vi "iWorx Drop Counter SubVI.vi"(4 "minimum drop delta (.05s)":dbl=0.01, 6 "# of Timestamps to store":i32=10, 7 "Reset count (f)":bool, 10 "Threshold (0V)":dbl, 11 "waveform in":waveform(dbl)) -> (0 "Rising Edge Times":timestamp[](array[timestamp]), 1 "Avg Drops Rate":dbl format="%.2f", 2 "Instantaneous Drop Rate":dbl format="%.2f", 3 "Drop Count":u32, 5 "Elasped Time (s)":dbl)   [LabVIEW 2012]
doc: "This subVI is designed to work with the iWorx Drop Coutner. It takes in a waveform from the sensor and records timestamps for each rising edge, and returns a count of the number of drops detected."
uses:
  <vilib>/ptbypt/NI_PtbyPt.lvlib
panel:
  out "drop delta":dbl[](array[numeric])
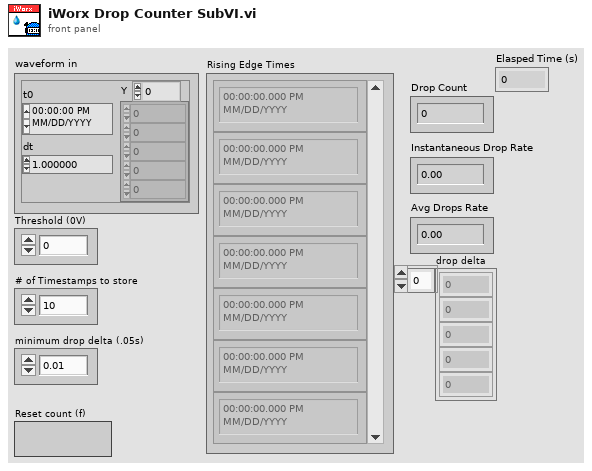
[diagram p1: front panel]
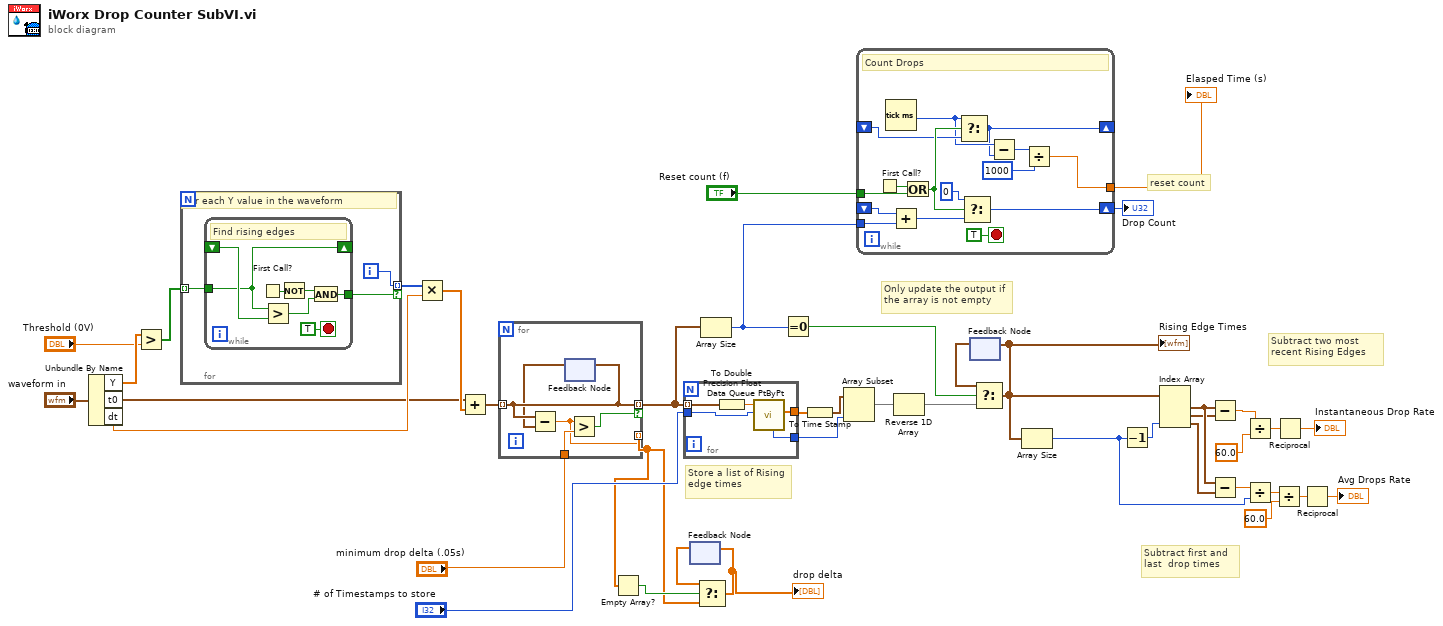
[diagram p0: block diagram]
diagram:
  # "Subtract first and last  drop times"
  # "reset count"
  # "Subtract two most recent Rising Edges"
  # "Only update the output if the array is not empty"
  # "Store a list of Rising edge times"
  n1 = Unbundle By Name("waveform in") -> ("Y"=w32:dbl[], "t0"=w39:timestamp, "dt"=w41:dbl)
  n2 = Greater?(x=w32, y="Threshold (0V)") -> (0:w30:bool[])
  n3 = for {
    tunnel: [w45] -> w42 mode=indexing if=w43
    tunnel: w30 -> [w44] mode=indexing
    i -> [w45]
    # "For each Y value in the waveform"
    n4 = while {
      shift-right: [w47] -> _
      shift-left: _ -> [w51]
      tunnel: w44 -> [w47]
      tunnel: [w46] -> w43
      stop <- TRUE stop-if-true
      # "Find rising edges"
      n5 = First Call?() -> (First Call?: T/F=w48:bool)
      n6 = Greater?(x=w47, y=w51) -> (0:w52:bool)
      n7 = Not(x=w48) -> (.not. x?=w49:bool)
      n8 = And(x=w49, y=w52) -> (x .and. y?=w46:bool)
    }
  }
  n9 = Multiply(x=w42, y=w41) -> (x*y=w40:dbl[])
  n10 = Add(x=w39, y=w40) -> (x+y=w14:timestamp[])
  n11 = for {
    tunnel: w14 -> [w54] mode=indexing
    tunnel: [w54] -> w12 mode=indexing if=w56
    tunnel: "minimum drop delta (.05s)" -> [w57]
    tunnel: [w55] -> w8 mode=indexing
    n12 = feedback #1() -> (w53:timestamp)  [unwired: 1 in]
    n13 = Subtract(x=w54, y=w53) -> (x-y=w55:dbl)
    n14 = feedback-in #1(w54) -> ()
    n15 = Greater?(x=w55, y=w57) -> (0:w56:bool)
  }
  n16 = Empty Array?(array=w8) -> (empty?=w10:bool)
  n17 = for {
    tunnel: w12 -> [w61] mode=indexing
    tunnel: "# of Timestamps to store" -> [w60]
    tunnel: [w59] -> w6
    tunnel: [w58] -> w4
    n18 = To Double Precision Float(number=w61) -> (double precision float=w62:dbl)
    n19 = call <vilib>:"Data Queue PtByPt.vi"("sample length"=w60, "input data point"=w62) -> ("Current Queue"=w59:dbl[], "current length"=w58:i32)  [unwired: 5 in, 3 out]
  }
  n20 = feedback #2() -> (w9:dbl[])  [unwired: 1 in]
  n21 = Select(t=w9, s=w10, f=w8) -> (s? t:f=w7:dbl[])
  "drop delta" <- w7
  n22 = feedback-in #2(w7) -> ()
  n23 = Array Size(array=w12) -> (size(s)=w37:i32)
  n24 = Equal To 0?(x=w37) -> (x = 0?=w35:bool)
  n25 = To Time Stamp(1:w6) -> (0:w5:timestamp[])
  n26 = Array Subset(array=w5, length=w4) -> (w3:timestamp[])  [unwired: 1 in]
  n27 = while {
    shift-right: [w73] -> w36
    shift-left: _ -> [w74]
    tunnel: w37 -> [w72]
    tunnel: "Reset count (f)" -> [w70]
    shift-right: [w63] -> _
    shift-left: _ -> [w68]
    tunnel: [w64] -> w1
    stop <- TRUE stop-if-true
    # "Count Drops"
    n28 = First Call?() -> (First Call?: T/F=w76:bool)
    n29 = Tick Count (ms)() -> (millisecond timer value=w67:u32)
    n30 = Add(x=w74, y=w72) -> (x+y=w71:u32)
    n31 = Or(x=w76, y=w70) -> (x .or. y?=w69:bool)
    n32 = Select(t=w67, s=w69, f=w68) -> (s? t:f=w63:u32)
    n33 = Select(t=u32 0, s=w69, f=w71) -> (s? t:f=w73:u32)
    n34 = Subtract(x=w67, y=w63) -> (x-y=w66:u32)
    n35 = Divide(x=w66, y=u32 1000) -> (x/y=w64:dbl)
  }
  "Drop Count" <- w36
  "Elasped Time (s)" <- w1
  n36 = Reverse 1D Array(array=w3) -> (reversed array=w2:timestamp[])
  n37 = feedback #3() -> (w13:timestamp[])  [unwired: 1 in]
  n38 = Select(t=w13, s=w35, f=w2) -> (s? t:f=w15:timestamp[])
  "Rising Edge Times" <- w15
  n39 = feedback-in #3(w15) -> ()
  n40 = Array Size(array=w15) -> (size(s)=w25:i32)
  n41 = Decrement(x=w25) -> (x-1=w21:i32)
  n42 = Index Array(array=w15, index #3=w21) -> (element #1=w22:timestamp, element #2=w18:timestamp, element #3=w23:timestamp)  [unwired: 2 in]
  n43 = Subtract(x=w22, y=w18) -> (x-y=w19:dbl)
  n44 = Subtract(x=w22, y=w23) -> (x-y=w24:dbl)
  n45 = Divide(x=w19, y=60.0) -> (x/y=w16:dbl)
  n46 = Divide(x=w24, y=w25) -> (x/y=w27:dbl)
  n47 = Divide(x=w27, y=60.0) -> (x/y=w28:dbl)
  n48 = Reciprocal(x=w16) -> (1/x=→"Instantaneous Drop Rate":dbl)
  n49 = Reciprocal(x=w28) -> (1/x=→"Avg Drops Rate":dbl)
